vi "Nanosleep Absolute (timespec).vi"(8 "error in (no error)":errorcluster, 10 "clock id (realtime)":T1, 11 "sleep until (timespec)":cluster{"sec":u64, "nsec":u64}) -> (0 "error out":errorcluster, 3 "current time (timspec)":cluster{"sec":u64, "nsec":u64})   [LabVIEW 2013, in "Linux RT Utilities.lvlib"]
doc: "This VI sleeps the calling thread until the specified absolute time has been reached.\n\nThe provided absolute time is evaluated against the selected clock. To create an appropriate absolute timeout, use the Get Clock Time VI to first get the current time on the specified clock, and then offset the current time by the desired sleep duration."
uses:
  Linux RT Utilities.lvlib
  Controls/Public/C Enums/clockid_t.ctl
  Controls/Public/nanosleep flags.ctl
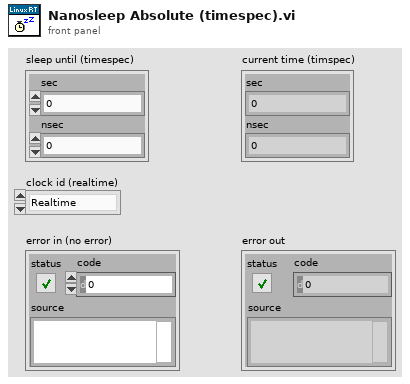
[diagram p1: front panel]
types:
  T1 = typedef "Linux RT Utilities.lvlib/clockid_t.ctl" = enum16{"Realtime", "Monotonic"}
  T2 = typedef "Linux RT Utilities.lvlib/nanosleep flags.ctl" = enum16{"Relative Time", "Absolute Time"}
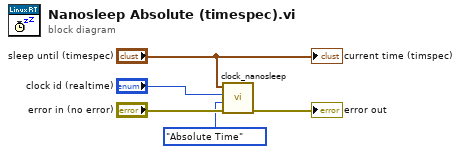
[diagram p0: block diagram]
diagram:
  n1 = call "clock_nanosleep.vi"("error in (no error)"="error in (no error)", "flags"=nanosleep_flags."Absolute Time", "clockid_t"="clock id (realtime)", "request"="sleep until (timespec)") -> ("error out"=→"error out":errorcluster)  [unwired: 6 in, 1 out]
  "current time (timspec)" <- "sleep until (timespec)"
